vi "getFilePaths.vi"(8 "Error In":errorcluster) -> (0 "Error Out":errorcluster, 3 "Application Path Cluster":T1)   [LabVIEW 2018]
uses:
  controls/pathCluster.ctl
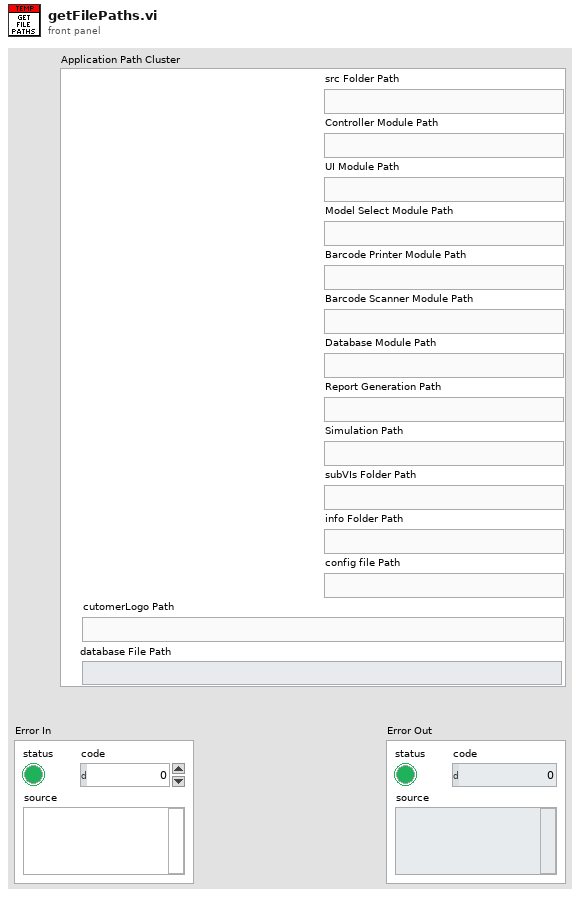
[diagram p1: front panel]
types:
  T1 = typedef "pathCluster.ctl" = cluster{"src Folder Path":path, "Controller Module Path":path, "UI Module Path":path, "Model Select Module Path":path, "Barcode Printer Module Path":path, "Barcode Scanner Module Path":path, "Database Module Path":path, "Report Generation Path":path, "Simulation Path":path, "subVIs Folder Path":path, "info Folder Path":path, "config file Path":path, "cutomerLogo Path":path, "database File Path":path}
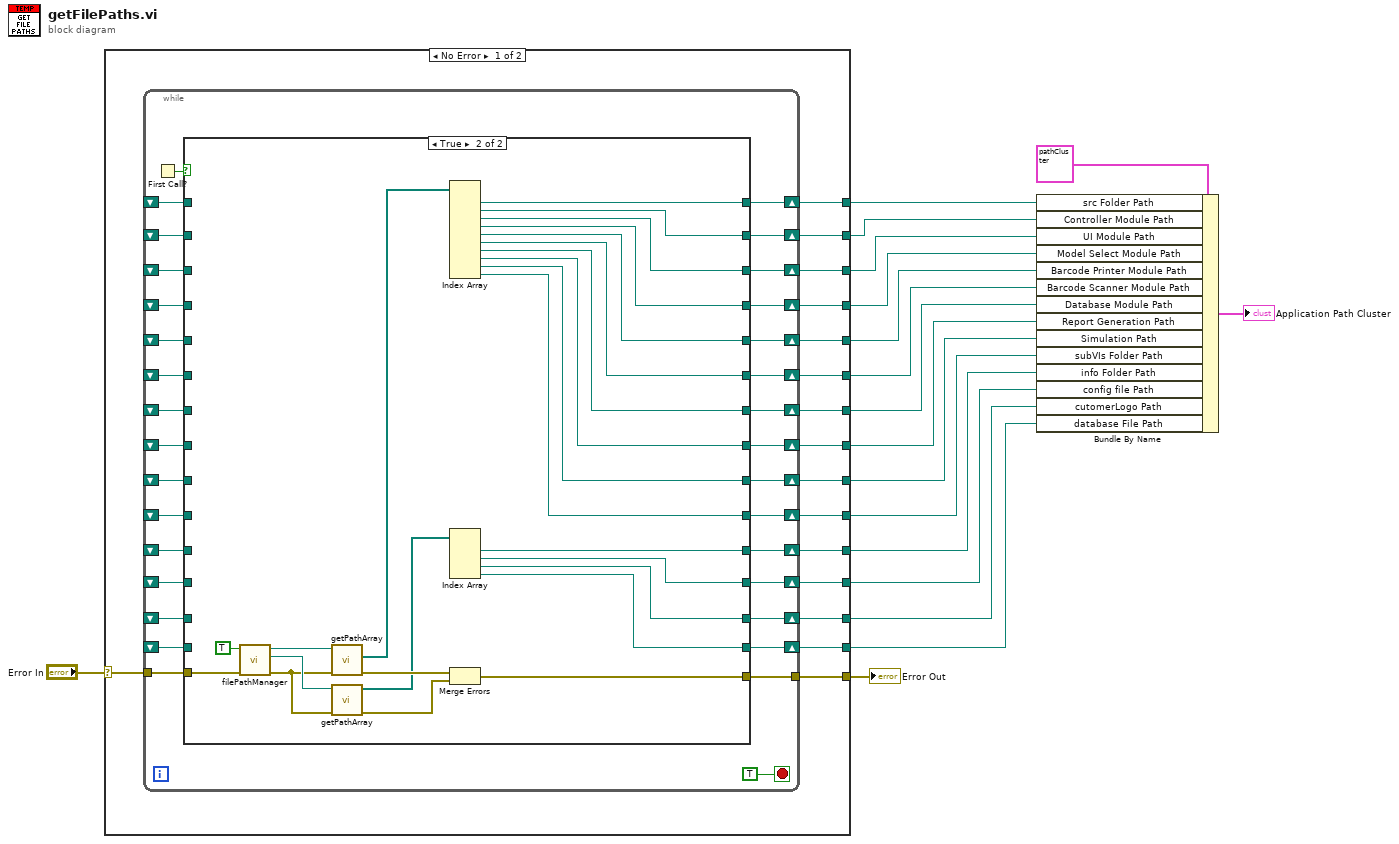
[diagram p0: block diagram]
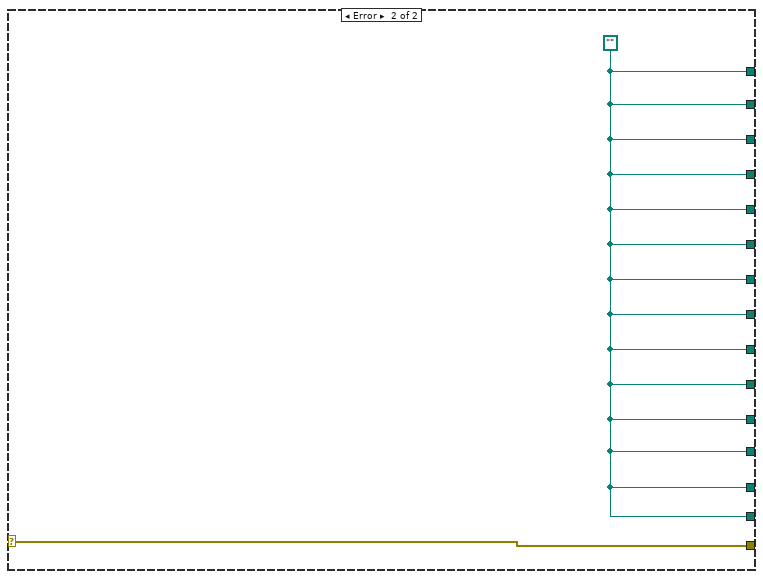
[diagram p3: hidden frame]
diagram:
  n1 = case shown="No Error" "Error In" {
    selector: "Error In" -> [w34 w107]
    tunnel: [w33 w107] -> w2
    tunnel: [w32 w106] -> w17
    tunnel: [w31 w106] -> w16
    tunnel: [w30 w106] -> w14
    tunnel: [w29 w106] -> w13
    tunnel: [w28 w106] -> w11
    tunnel: [w27 w106] -> w10
    tunnel: [w26 w106] -> w9
    tunnel: [w25 w106] -> w8
    tunnel: [w24 w106] -> w7
    tunnel: [w23 w106] -> w6
    tunnel: [w22 w106] -> w5
    tunnel: [w21 w106] -> w4
    tunnel: [w20 w106] -> w12
    tunnel: [w19 w106] -> w1
    frame No Error {
      n2 = while {
        tunnel: w34 -> [w66]
        tunnel: [w65] -> w33
        shift-right: [w63] -> w32
        shift-left: _ -> [w61]
        shift-right: [w62] -> w31
        shift-left: _ -> [w60]
        shift-right: [w59] -> w30
        shift-left: _ -> [w58]
        shift-right: [w57] -> w29
        shift-left: _ -> [w56]
        shift-right: [w54] -> w28
        shift-left: _ -> [w46]
        shift-right: [w53] -> w27
        shift-left: _ -> [w45]
        shift-right: [w52] -> w26
        shift-left: _ -> [w44]
        shift-right: [w51] -> w25
        shift-left: _ -> [w43]
        shift-right: [w50] -> w24
        shift-left: _ -> [w42]
        shift-right: [w49] -> w23
        shift-left: _ -> [w41]
        shift-right: [w55] -> w22
        shift-left: _ -> [w40]
        shift-right: [w48] -> w21
        shift-left: _ -> [w39]
        shift-right: [w47] -> w20
        shift-left: _ -> [w38]
        shift-right: [w36] -> w19
        shift-left: _ -> [w35]
        stop <- TRUE stop-if-true
        n3 = First Call?() -> (First Call?: T/F=w64:bool)
        n4 = case shown="True" w64 {
          tunnel: w66 -> [w81 w105]
          tunnel: [w81 w99] -> w65
          tunnel: [w80 w95] -> w63
          tunnel: [w79 w94] -> w62
          tunnel: w61 -> [w80 _]
          tunnel: w60 -> [w79 _]
          tunnel: [w78 w93] -> w59
          tunnel: w58 -> [w78 _]
          tunnel: [w77 w92] -> w57
          tunnel: w56 -> [w77 _]
          tunnel: [w70 w85] -> w55
          tunnel: [w76 w91] -> w54
          tunnel: [w75 w90] -> w53
          tunnel: [w74 w89] -> w52
          tunnel: [w73 w88] -> w51
          tunnel: [w72 w87] -> w50
          tunnel: [w71 w86] -> w49
          tunnel: [w69 w84] -> w48
          tunnel: [w68 w83] -> w47
          tunnel: w46 -> [w76 _]
          tunnel: w45 -> [w75 _]
          tunnel: w44 -> [w74 _]
          tunnel: w43 -> [w73 _]
          tunnel: w42 -> [w72 _]
          tunnel: w41 -> [w71 _]
          tunnel: w40 -> [w70 _]
          tunnel: w39 -> [w69 _]
          tunnel: w38 -> [w68 _]
          tunnel: [w67 w82] -> w36
          tunnel: w35 -> [w67 _]
          frame False {
          }
          frame True {
            n5 = call "filePathManager.vi"("Error In"=w105, "First Call?"=TRUE) -> ("Error Out"=w100:errorcluster, "info File Path"=w101:path, "src File Path"=w103:path)  [unwired: 7 in]
            n6 = call "getPathArray.vi"("Error In"=w100, "File Path"=w103) -> ("Error Out"=w102:errorcluster, "Folder Path Array"=w97:path[])  [unwired: 7 in, 1 out]
            n7 = call "getPathArray.vi"("Error In"=w100, "File Path"=w101) -> ("Error Out"=w98:errorcluster, "File Path Array"=w96:path[])  [unwired: 7 in, 1 out]
            n8 = Index Array(array=w97) -> (element #1=w95:path, element #2=w94:path, element #3=w93:path, element #4=w92:path, element #5=w91:path, element #6=w90:path, element #7=w89:path, element #8=w88:path, element #9=w87:path, element #10=w86:path)  [unwired: 10 in]
            n9 = Index Array(array=w96) -> (element #1=w85:path, element #2=w84:path, element #3=w83:path, element #4=w82:path)  [unwired: 4 in]
            n10 = Merge Errors(w102, w98) -> (w99:errorcluster)
          }
        }
      }
    }
    frame Error {
      w106 = path ""
    }
  }
  "Error Out" <- w2
  n11 = Bundle By Name(cluster=T1 {"src Folder Path"=path "", "Controller Module Path"=path "", "UI Module Path"=path "", "Model Select Module Path"=path "", "Barcode Printer Module Path"=path "", "Barcode Scanner Module Path"=path "", "Database Module Path"=path "", "Report Generation Path"=path "", "Simulation Path"=path "", "subVIs Folder Path"=path "", "info Folder Path"=path "", "config file Path"=path "", "cutomerLogo Path"=path "", "database File Path"=path ""} ("Path Cluster"), "src Folder Path"=w17, "Controller Module Path"=w16, "UI Module Path"=w14, "Model Select Module Path"=w13, "Barcode Printer Module Path"=w11, "Barcode Scanner Module Path"=w10, "Database Module Path"=w9, "Report Generation Path"=w8, "Simulation Path"=w7, "subVIs Folder Path"=w6, "info Folder Path"=w5, "config file Path"=w4, "cutomerLogo Path"=w12, "database File Path"=w1) -> (→"Application Path Cluster":T1)
